vi "TeleopStateMachine.vi"(4 "PegAim":bool, 6 "GearAim":bool, 8 "Target Data":T2, 9 "Right Joystick":dbl, 10 "Left Joystick":dbl) -> (3 "TeleState":T1)   [LabVIEW 2016]
uses:
  TeleopStates.ctl
  Drive Base Class/DriveBase.lvclass
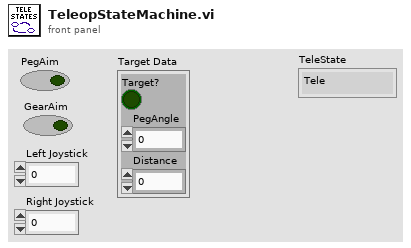
[diagram p1: front panel]
types:
  T1 = typedef "TeleopStates.ctl" = enum16{"Tele", "PegAim", "GearAim", "PegForward", "GearForward", "Place", "Back"}
  T2 = cluster{"Target?":bool, "PegAngle":dbl, "Distance":dbl}
  T3 = cluster{"Lower X":dbl, "Lower Y":dbl, "Upper X":dbl, "Upper Y":dbl, "Lower Limit":dbl, "Upper Limit":dbl}
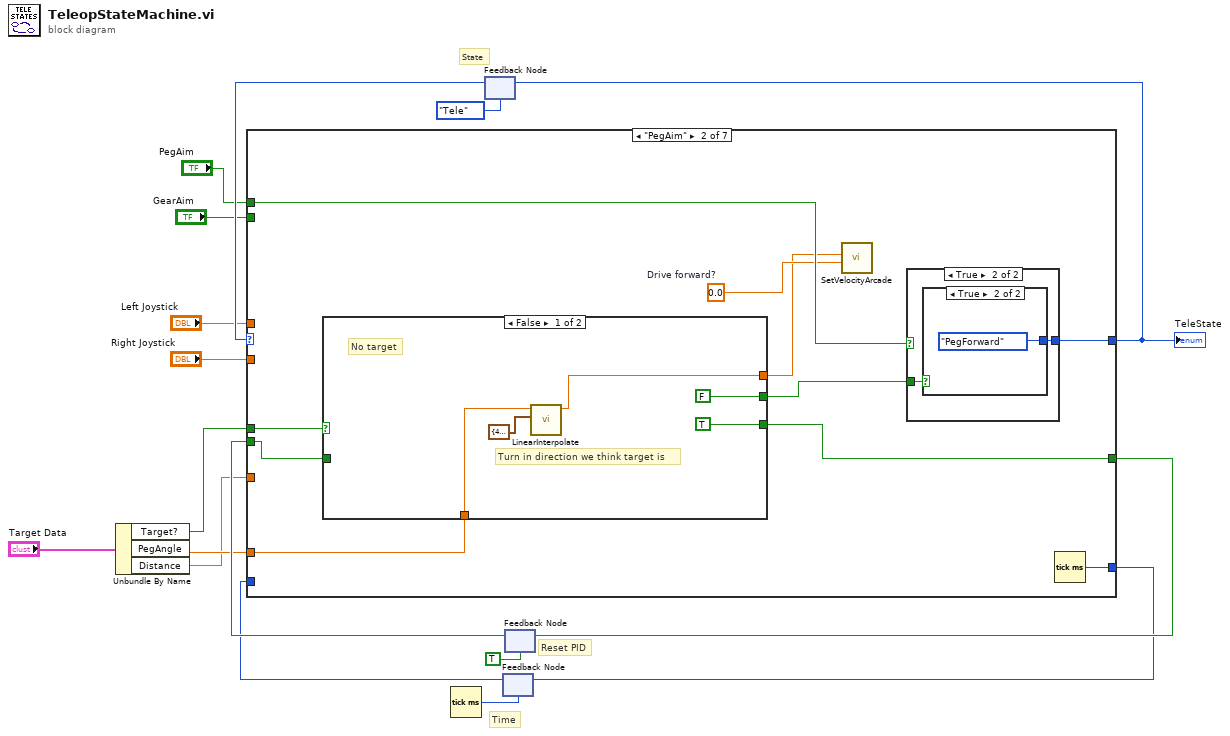
[diagram p0: block diagram]
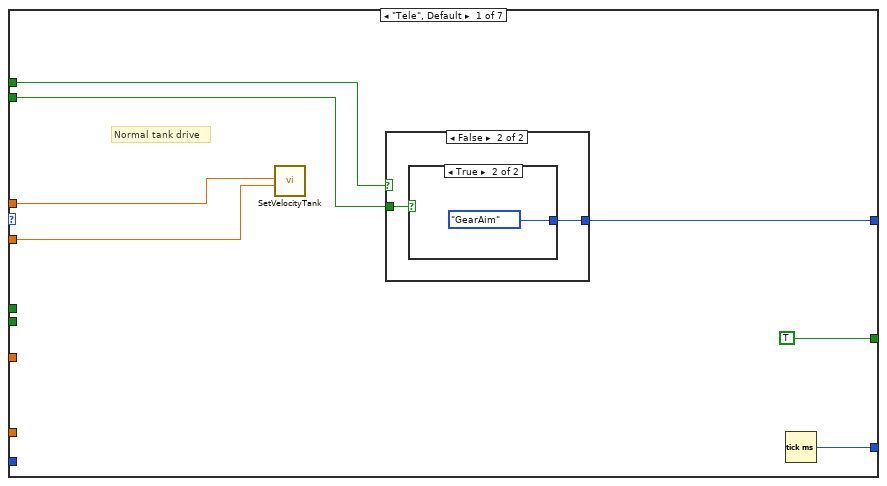
[diagram p2: hidden frame]
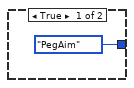
[diagram p3: hidden frame]
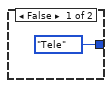
[diagram p4: hidden frame]
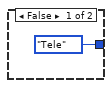
[diagram p5: hidden frame]
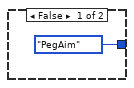
[diagram p6: hidden frame]
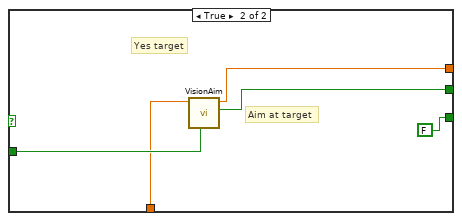
[diagram p7: hidden frame]
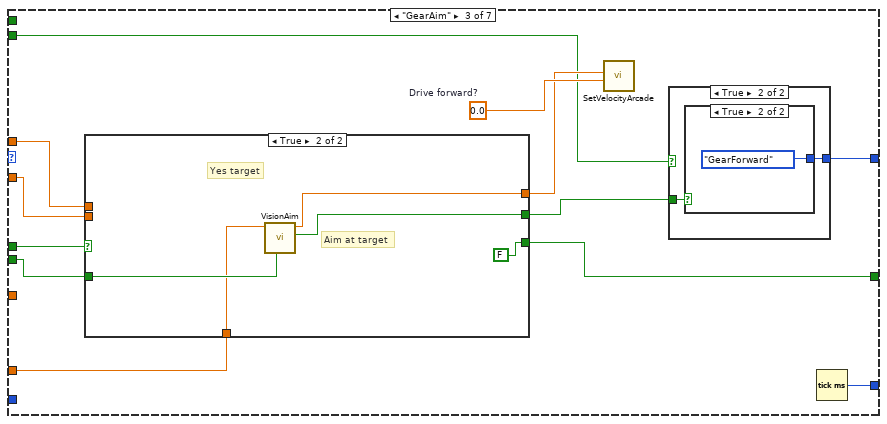
[diagram p8: hidden frame]
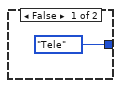
[diagram p9: hidden frame]
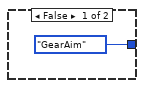
[diagram p10: hidden frame]
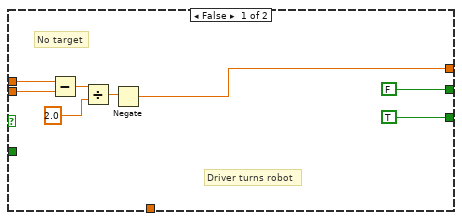
[diagram p11: hidden frame]
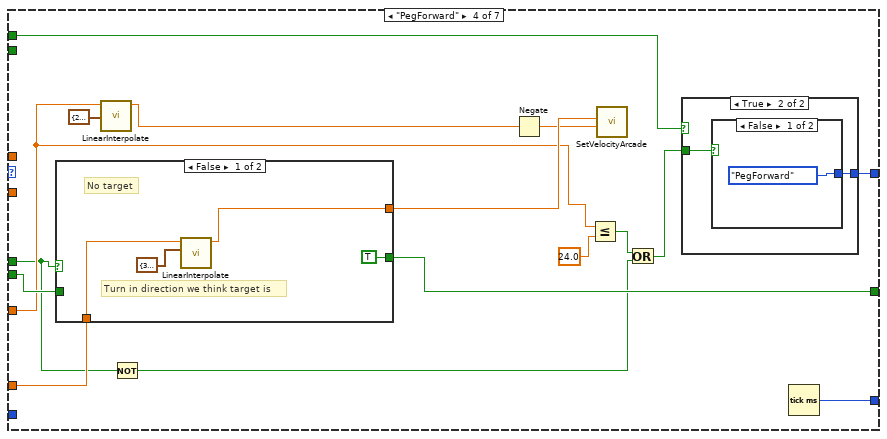
[diagram p12: hidden frame]
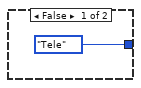
[diagram p13: hidden frame]
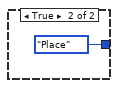
[diagram p14: hidden frame]
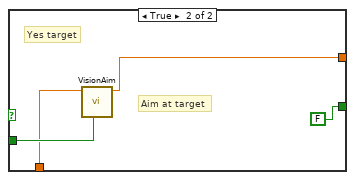
[diagram p15: hidden frame]
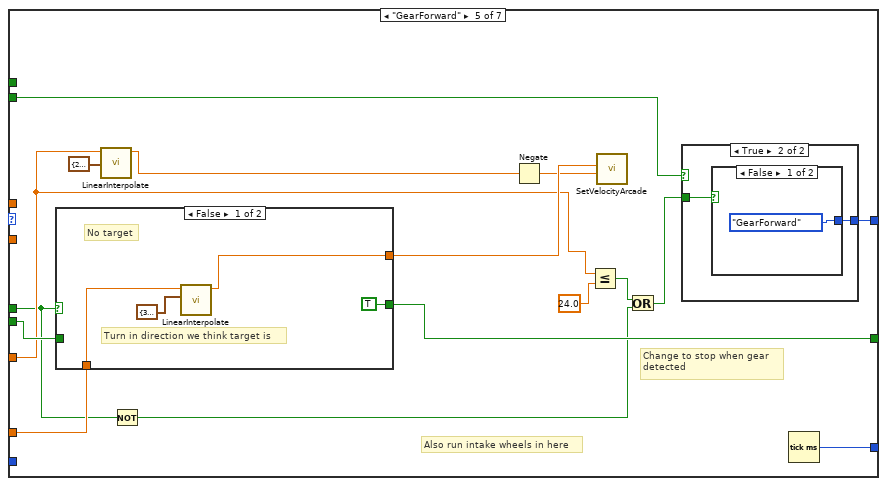
[diagram p16: hidden frame]
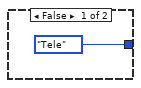
[diagram p17: hidden frame]
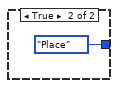
[diagram p18: hidden frame]
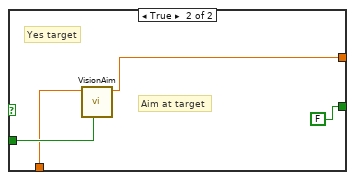
[diagram p19: hidden frame]
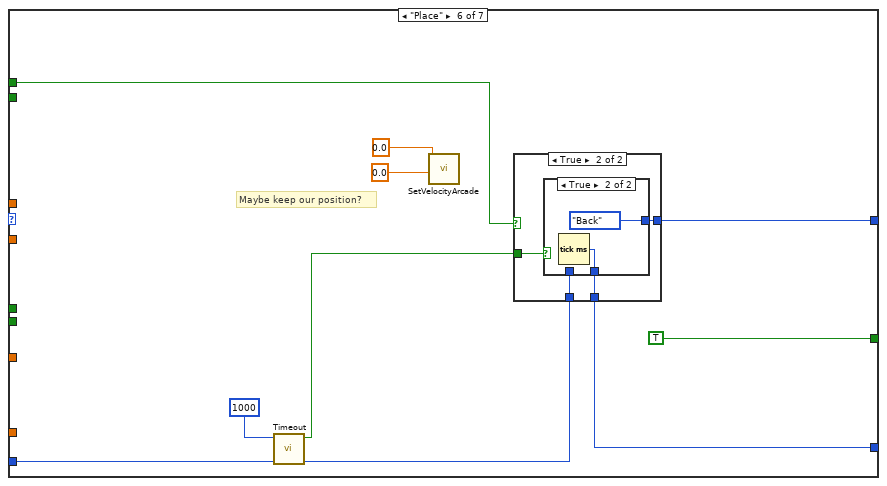
[diagram p20: hidden frame]
diagram:
  # "State"
  # "Reset PID"
  # "Time"
  n1 = Unbundle By Name("Target Data") -> ("Target?"=w5:bool, "PegAngle"=w4:dbl, "Distance"=w3:dbl)
  n2 = Tick Count (ms)() -> (millisecond timer value=w10:u32)
  n3 = feedback #1(TeleopStates."Tele" ("PlaceGearStates")) -> (w14:T1)
  n4 = feedback #2(w10) -> (w11:u32)
  n5 = feedback #3(TRUE ("x .and. y?")) -> (w12:bool)
  n6 = case shown="\"PegAim\"" w14 {
    tunnel: [TRUE ("x .and. y?") w39 w66 w100 w129 TRUE ("x .and. y?") TRUE ("x .and. y?")] -> w16
    tunnel: [w23 w36 w63 w98 w127 w152 w172] -> w13
    tunnel: w12 -> [_ w38 w65 w99 w128 _ _]
    tunnel: w5 -> [_ w37 w64 w86 w116 _ _]
    tunnel: "PegAim" -> [w22 w34 _ w97 _ w151 w171]
    tunnel: w11 -> [_ _ _ _ _ w148 w169]
    tunnel: [w21 w33 w61 w91 w121 w144 w166] -> w15
    tunnel: w4 -> [_ w32 w60 w90 w120 _ _]
    tunnel: "Left Joystick" -> [w18 _ w57 _ _ _ _]
    tunnel: "Right Joystick" -> [w19 _ w56 _ _ _ _]
    tunnel: w3 -> [_ _ _ w89 w119 _ _]
    tunnel: "GearAim" -> [w20 _ w55 _ w114 _ _]
    frame "Tele", Default {
      # "Normal tank drive"
      n7 = call "SetVelocityTank.vi"("rightVelocitySetpointInput"=w19, "leftVelocitySetpointInput"=w18) -> ()  [unwired: 9 in, 1 out]
      n8 = case shown="False" w22 {
        tunnel: [TeleopStates."PegAim" ("PlaceGearStates") w27] -> w23
        tunnel: w20 -> [_ w26]
        frame True {
        }
        frame False {
          n9 = case shown="True" w26 {
            tunnel: [TeleopStates."Tele" ("PlaceGearStates") TeleopStates."GearAim" ("PlaceGearStates")] -> w27
            frame False {
            }
            frame True {
            }
          }
        }
      }
      n10 = Tick Count (ms)() -> (millisecond timer value=w21:u32)
    }
    frame "PegAim" {
      w31 = 0.0  # Drive forward?
      n11 = case shown="False" w37 {
        tunnel: [w48 w54] -> w30
        tunnel: [TRUE ("x .and. y?") FALSE ("x .and. y?")] -> w39
        tunnel: w38 -> [_ w52]
        tunnel: [FALSE ("In Range") w51] -> w35
        tunnel: w32 -> [w46 w50]
        frame False {
          # "Turn in direction we think target is"
          # "No target"
          n12 = call "LinearInterpolate.vi"("Config"=T3 {"Lower X"=45.0, "Lower Y"=0.5, "Upper X"=100.0, "Upper Y"=0.8, "Lower Limit"=0.5, "Upper Limit"=0.85}, "Value"=w46) -> ("Ouput"=w48:dbl)  [unwired: 9 in]
        }
        frame True {
          # "Yes target"
          # "Aim at target"
          n13 = call "VisionAim.vi"("Reset PID"=w52, "Angle"=w50) -> ("In Range"=w51:bool, "Turn Amount"=w54:dbl)  [unwired: 8 in]
        }
      }
      n14 = call "SetVelocityArcade.vi"("Y Axis"=w31, "X Axis"=w30) -> ()  [unwired: 9 in, 1 out]
      n15 = case shown="True" w34 {
        tunnel: [TeleopStates."Tele" ("PlaceGearStates") w41] -> w36
        tunnel: w35 -> [_ w42]
        frame False {
        }
        frame True {
          n16 = case shown="True" w42 {
            tunnel: [TeleopStates."PegAim" ("PlaceGearStates") TeleopStates."PegForward" ("PlaceGearStates")] -> w41
            frame False {
            }
            frame True {
            }
          }
        }
      }
      n17 = Tick Count (ms)() -> (millisecond timer value=w33:u32)
    }
    frame "GearAim" {
      w59 = 0.0  # Drive forward?
      n18 = case shown="True" w64 {
        tunnel: [w72 w84] -> w58
        tunnel: [TRUE ("x .and. y?") FALSE ("x .and. y?")] -> w66
        tunnel: w65 -> [_ w82]
        tunnel: [FALSE ("In Range") w81] -> w62
        tunnel: w60 -> [_ w80]
        tunnel: w57 -> [w77 _]
        tunnel: w56 -> [w76 _]
        frame False {
          # "Driver turns robot"
          # "No target"
          n19 = Subtract(x=w77, y=w76) -> (x-y=w75:dbl)
          n20 = Divide(x=w75, y=2.0) -> (x/y=w73:dbl)
          n21 = Negate(x=w73) -> (-x=w72:dbl)
        }
        frame True {
          # "Yes target"
          # "Aim at target"
          n22 = call "VisionAim.vi"("Reset PID"=w82, "Angle"=w80) -> ("In Range"=w81:bool, "Turn Amount"=w84:dbl)  [unwired: 8 in]
        }
      }
      n23 = call "SetVelocityArcade.vi"("Y Axis"=w59, "X Axis"=w58) -> ()  [unwired: 9 in, 1 out]
      n24 = case shown="True" w55 {
        tunnel: [TeleopStates."Tele" ("PlaceGearStates") w68] -> w63
        tunnel: w62 -> [_ w69]
        frame False {
        }
        frame True {
          n25 = case shown="True" w69 {
            tunnel: [TeleopStates."GearAim" ("PlaceGearStates") TeleopStates."GearForward" ("PlaceGearStates")] -> w68
            frame False {
            }
            frame True {
            }
          }
        }
      }
      n26 = Tick Count (ms)() -> (millisecond timer value=w61:u32)
    }
    frame "PegForward" {
      n27 = case shown="False" w86 {
        tunnel: [w108 w113] -> w95
        tunnel: [TRUE ("x .and. y?") FALSE ("x .and. y?")] -> w100
        tunnel: w99 -> [_ w111]
        tunnel: w90 -> [w106 w110]
        frame False {
          # "No target"
          # "Turn in direction we think target is"
          n28 = call "LinearInterpolate.vi"("Config"=T3 {"Lower X"=30.0, "Lower Y"=0.6, "Upper X"=100.0, "Upper Y"=0.9, "Lower Limit"=0.6, "Upper Limit"=0.9}, "Value"=w106) -> ("Ouput"=w108:dbl)  [unwired: 9 in]
        }
        frame True {
          # "Yes target"
          # "Aim at target"
          n29 = call "VisionAim.vi"("Reset PID"=w111, "Angle"=w110) -> ("Turn Amount"=w113:dbl)  [unwired: 8 in, 1 out]
        }
      }
      n30 = call "LinearInterpolate.vi"("Config"=T3 {"Lower X"=24.0, "Lower Y"=0.48, "Upper X"=65.0, "Upper Y"=0.8, "Lower Limit"=0.45, "Upper Limit"=0.75}, "Value"=w89) -> ("Ouput"=w92:dbl)  [unwired: 9 in]
      n31 = Not(x=w86) -> (.not. x?=w85:bool)
      n32 = Negate(x=w92) -> (-x=w94:dbl)
      n33 = Less Or Equal?(x=w89, y=24.0) -> (x <= y?=w88:bool)
      n34 = call "SetVelocityArcade.vi"("Y Axis"=w94, "X Axis"=w95) -> ()  [unwired: 9 in, 1 out]
      n35 = Or(x=w88, y=w85) -> (x .or. y?=w87:bool)
      n36 = case shown="True" w97 {
        tunnel: [TeleopStates."Tele" ("PlaceGearStates") w102] -> w98
        tunnel: w87 -> [_ w103]
        frame False {
        }
        frame True {
          n37 = case shown="False" w103 {
            tunnel: [TeleopStates."PegForward" ("PlaceGearStates") TeleopStates."Place" ("PlaceGearStates")] -> w102
            frame False {
            }
            frame True {
            }
          }
        }
      }
      n38 = Tick Count (ms)() -> (millisecond timer value=w91:u32)
    }
    frame "GearForward" {
      # "Also run intake wheels in here"
      # "Change to stop when gear\ndetected"
      n39 = case shown="False" w116 {
        tunnel: [w137 w142] -> w125
        tunnel: [TRUE ("x .and. y?") FALSE ("x .and. y?")] -> w129
        tunnel: w128 -> [_ w140]
        tunnel: w120 -> [w135 w139]
        frame False {
          # "No target"
          # "Turn in direction we think target is"
          n40 = call "LinearInterpolate.vi"("Config"=T3 {"Lower X"=30.0, "Lower Y"=0.6, "Upper X"=100.0, "Upper Y"=0.9, "Lower Limit"=0.6, "Upper Limit"=0.9}, "Value"=w135) -> ("Ouput"=w137:dbl)  [unwired: 9 in]
        }
        frame True {
          # "Yes target"
          # "Aim at target"
          n41 = call "VisionAim.vi"("Reset PID"=w140, "Angle"=w139) -> ("Turn Amount"=w142:dbl)  [unwired: 8 in, 1 out]
        }
      }
      n42 = call "LinearInterpolate.vi"("Config"=T3 {"Lower X"=24.0, "Lower Y"=0.48, "Upper X"=65.0, "Upper Y"=0.8, "Lower Limit"=0.45, "Upper Limit"=0.75}, "Value"=w119) -> ("Ouput"=w122:dbl)  [unwired: 9 in]
      n43 = Not(x=w116) -> (.not. x?=w115:bool)
      n44 = Negate(x=w122) -> (-x=w124:dbl)
      n45 = Less Or Equal?(x=w119, y=24.0) -> (x <= y?=w118:bool)
      n46 = call "SetVelocityArcade.vi"("Y Axis"=w124, "X Axis"=w125) -> ()  [unwired: 9 in, 1 out]
      n47 = Or(x=w118, y=w115) -> (x .or. y?=w117:bool)
      n48 = case shown="True" w114 {
        tunnel: [TeleopStates."Tele" ("PlaceGearStates") w131] -> w127
        tunnel: w117 -> [_ w132]
        frame False {
        }
        frame True {
          n49 = case shown="False" w132 {
            tunnel: [TeleopStates."GearForward" ("PlaceGearStates") TeleopStates."Place" ("PlaceGearStates")] -> w131
            frame False {
            }
            frame True {
            }
          }
        }
      }
      n50 = Tick Count (ms)() -> (millisecond timer value=w121:u32)
    }
    frame "Place" {
      # "Maybe keep our position?"
      n51 = call "Timeout.vi"("Start Time In"=w148, "Time Limit"=u32 1000) -> ("Start Time Out"=w143:u32, "Timeout"=w146:bool)  [unwired: 8 in]
      n52 = call "SetVelocityArcade.vi"("Y Axis"=0.0 ("Y axis value"), "X Axis"=0.0 ("X axis value")) -> ()  [unwired: 9 in, 1 out]
      n53 = case shown="True" w151 {
        tunnel: [TeleopStates."Tele" ("PlaceGearStates") w158] -> w152
        tunnel: w146 -> [_ w157]
        tunnel: [w153 w155] -> w144
        tunnel: w143 -> [_ w156]
        frame False {
          n54 = Tick Count (ms)() -> (millisecond timer value=w153:u32)
        }
        frame True {
          n55 = case shown="True" w157 {
            tunnel: [TeleopStates."Place" ("PlaceGearStates") TeleopStates."Back" ("PlaceGearStates")] -> w158
            tunnel: w156 -> [w159 _]
            tunnel: [w159 w161] -> w155
            frame False {
            }
            frame True {
              n56 = Tick Count (ms)() -> (millisecond timer value=w161:u32)
            }
          }
        }
      }
    }
    frame "Back" {
      # "Back up"
      n57 = call "Timeout.vi"("Start Time In"=w169, "Time Limit"=u32 500) -> ("Start Time Out"=w165:u32, "Timeout"=w167:bool)  [unwired: 8 in]
      n58 = call "SetVelocityArcade.vi"("Y Axis"=0.6 ("X axis value"), "X Axis"=0.0 ("Y axis value")) -> ()  [unwired: 9 in, 1 out]
      n59 = case shown="True" w171 {
        tunnel: [TeleopStates."Tele" ("PlaceGearStates") w178] -> w172
        tunnel: w167 -> [_ w177]
        tunnel: [w173 w175] -> w166
        tunnel: w165 -> [_ w176]
        frame False {
          n60 = Tick Count (ms)() -> (millisecond timer value=w173:u32)
        }
        frame True {
          n61 = case shown="True" w177 {
            tunnel: [TeleopStates."Back" ("PlaceGearStates") TeleopStates."Tele" ("PlaceGearStates")] -> w178
            tunnel: w176 -> [w179 _]
            tunnel: [w179 w181] -> w175
            frame False {
            }
            frame True {
              n62 = Tick Count (ms)() -> (millisecond timer value=w181:u32)
            }
          }
        }
      }
    }
  }
  "TeleState" <- w13
  n63 = feedback-in #1(w13) -> ()
  n64 = feedback-in #2(w15) -> ()
  n65 = feedback-in #3(w16) -> ()
